vi "Write Dark Color.vi"(8 "error in (no error)":errorcluster, 10 "Dark Color":u32(colorbox), 11 "BarCode in":refnum<class "BarCode.lvclass">) -> (0 "error out":errorcluster, 3 "BarCode out":refnum<class "BarCode.lvclass">)   [LabVIEW 2013, in "BarCodes.lvlib" / "BarCode.lvclass"]
doc: "Sets the dark color in the bar code. In typical bar codes, this is black."
uses:
  BarCode.lvclass
  BarCode.lvclass/BarCode.ctl
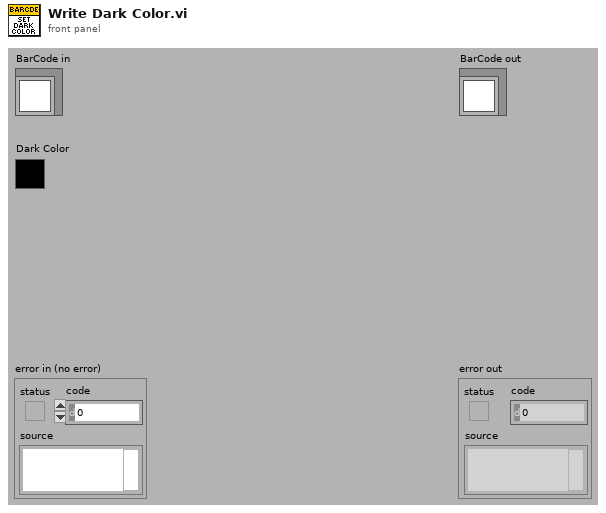
[diagram p1: front panel]
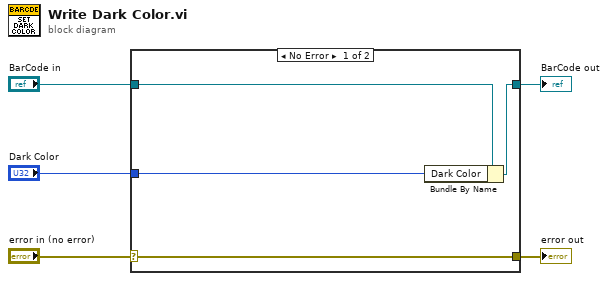
[diagram p0: block diagram]
diagram:
  n1 = case shown="No Error" "error in (no error)" {
    selector: "error in (no error)" -> [w9 w10]
    tunnel: [w9 w10] -> w4
    tunnel: [w7 w11] -> w2
    tunnel: "BarCode in" -> [w8 w11]
    tunnel: "Dark Color" -> [w6 _]
    frame No Error {
      n2 = Bundle By Name(cluster=w8, "Dark Color"=w6) -> (w7:refnum<class "BarCode.lvclass">)
    }
    frame Error {
    }
  }
  "error out" <- w4
  "BarCode out" <- w2
